vi "JAPCinitallTypes.vi"(8 "error in":errorcluster, 10 "Data Type":string, 11 "URL":string="VAC.VGHA_41677/PR") -> (0 "error out":errorcluster, 3 "JAPC out":refnum<class "JSubscribe.lvclass">)   [LabVIEW 2014]
uses:
  <userlib>/_RADE/RIO/JAPC/classes/JSubscribe/JSubscribe.lvclass
  <userlib>/_RADE/RIO/JAPC/classes/JSubscribe/openJAPCSubscribe.vi
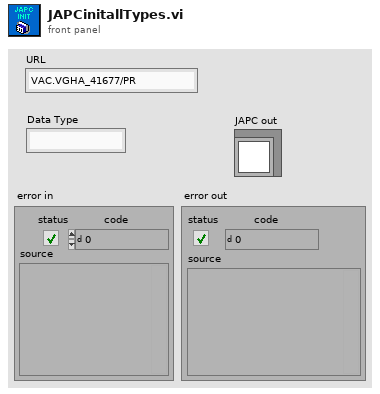
[diagram p1: front panel]
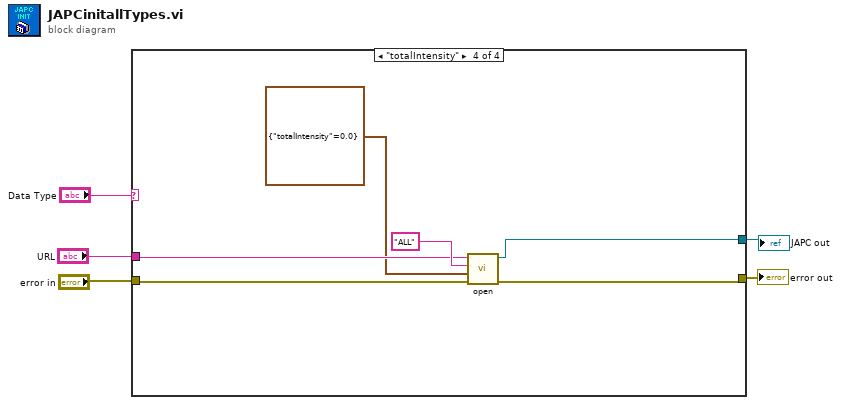
[diagram p0: block diagram]
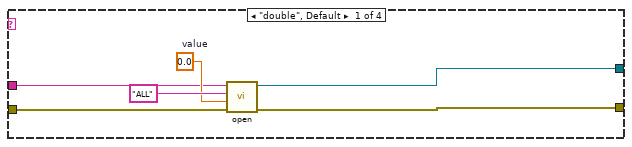
[diagram p2: hidden frame]
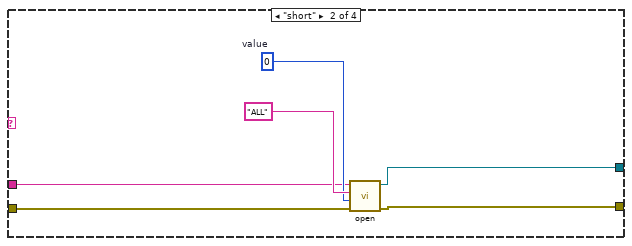
[diagram p3: hidden frame]
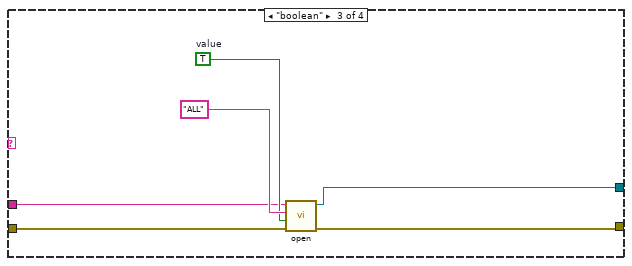
[diagram p4: hidden frame]
diagram:
  n1 = case shown="\"totalIntensity\"" "Data Type" {
    tunnel: "error in" -> [w8 w13 w20 w25]
    tunnel: [w9 w14 w19 w28] -> w2
    tunnel: "URL" -> [w7 w12 w21 w26]
    tunnel: [w6 w15 w18 w27] -> w1
    frame "double", Default {
      w10 = 0.0  # value
      n2 = call-poly <userlib>:"open.vi"("error in (no error)"=w8, "Data type"=w10, "Cycle"="ALL", "URL"=w7) -> ("error out"=w9:errorcluster, "Object out"=w6:refnum<class "JSubscribe.lvclass">)  [unwired: 6 in]
    }
    frame "short" {
      w16 = i16 0  # value
      n3 = call-poly <userlib>:"open.vi"("error in (no error)"=w13, "Data type"=w16, "Cycle"="ALL", "URL"=w12) -> ("error out"=w14:errorcluster, "Object out"=w15:refnum<class "JSubscribe.lvclass">)  [unwired: 6 in]
    }
    frame "boolean" {
      w22 = TRUE  # value
      n4 = call-poly <userlib>:"open.vi"("error in (no error)"=w20, "Data type"=w22, "Cycle"="ALL", "URL"=w21) -> ("error out"=w19:errorcluster, "Object out"=w18:refnum<class "JSubscribe.lvclass">)  [unwired: 6 in]
    }
    frame "totalIntensity" {
      n5 = call-poly <userlib>:"open.vi"("error in (no error)"=w25, "Data type"=cluster{"totalIntensity":sgl} {"totalIntensity"=0.0}, "Cycle"="ALL", "URL"=w26) -> ("error out"=w28:errorcluster, "Object out"=w27:refnum<class "JSubscribe.lvclass">)  [unwired: 6 in]
    }
  }
  "error out" <- w2
  "JAPC out" <- w1
